vi "set current as home.vi"(8 "error in (no error)":errorcluster, 9 "HOME":bool, 10 "DELAY (ms) in":u32, 11 "VISA Refnum in":refnum<visa-resource-name>) -> ()   [LabVIEW 2014]
doc: "this vi sets the current motor position as its home / default position"
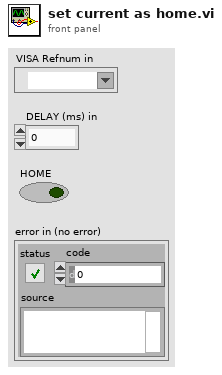
[diagram p1: front panel]
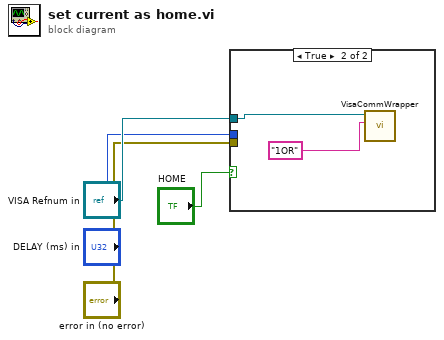
[diagram p0: block diagram]
diagram:
  n1 = case shown="True" "HOME" {
    tunnel: "DELAY (ms) in" -> [_ _]
    tunnel: "error in (no error)" -> [_ _]
    tunnel: "VISA Refnum in" -> [_ w6]
    frame False {
    }
    frame True {
      n2 = call <userlib>:"VisaCommWrapper.vi"("Command"="1OR", "VISA handle"=w6) -> ()  [unwired: 3 in, 5 out]
    }
  }
